vi "Rename Typedefs.vi"(8 "error in (no error)":errorcluster, 11 "ProjectItem in":refnum<class "ProjectItem.lvclass">) -> (0 "error out":errorcluster, 3 "ProjectItem out":refnum<class "ProjectItem.lvclass">)   [LabVIEW 2019, in "ProjectItem.lvclass"]
uses:
  ProjectItem.lvclass
  ProjectItem.lvclass/ProjectItem.ctl
panel:
  out "VI Names":string[](array[string])
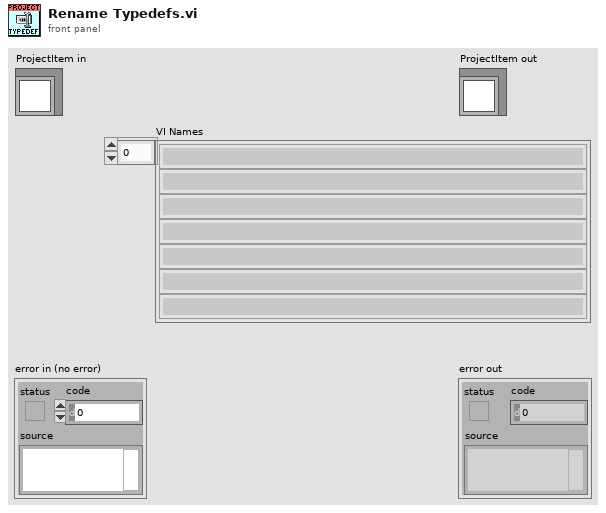
[diagram p1: front panel]
types:
  T1 = cluster{"Class":refnum<vi>, "DynamicVIs":refnum<vi>[], "StaticVIs":refnum<vi>[], "Controls":refnum<vi>[], "Name":string, "Icon":refnum<class "Icon.lvclass">, "Wire Foreground Color":u32}[]
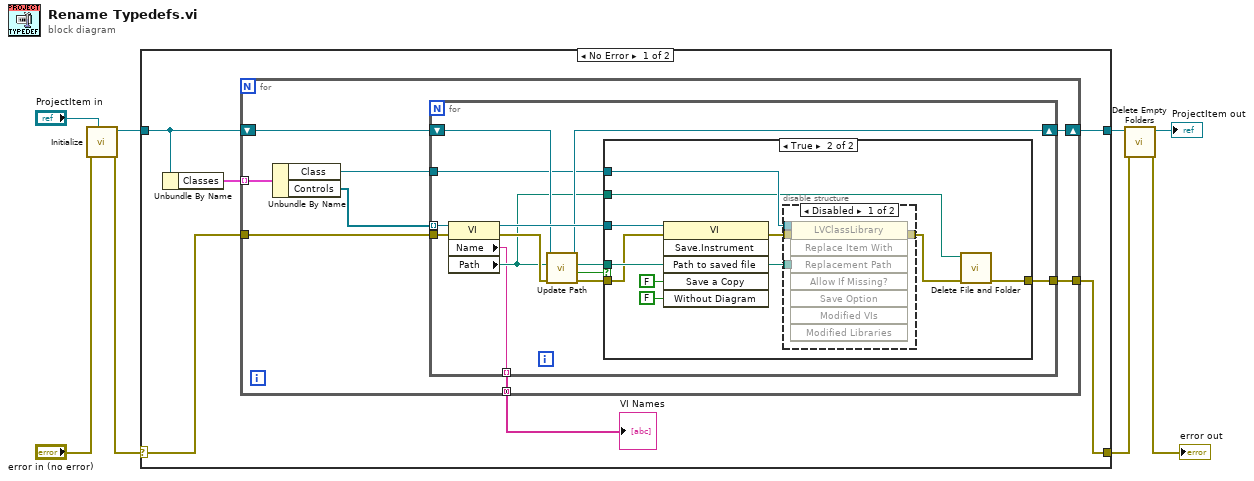
[diagram p0: block diagram]
diagram:
  n1 = call "Initialize.vi"("ProjectItem"="ProjectItem in", "error in (no error)"="error in (no error)") -> ("error out"=w5:errorcluster, "ProjectItem out"=w7:refnum<class "ProjectItem.lvclass">)  [unwired: 8 in]
  n2 = case shown="No Error" w5 {
    selector: w5 -> [w13 w53]
    tunnel: [w10 w53] -> w2
    tunnel: [w14 w52] -> w4
    tunnel: w7 -> [w11 w52]
    frame No Error {
      n3 = Unbundle By Name(w11) -> ("Classes"=w12:T1)
      n4 = for {
        tunnel: w13 -> [w22]
        shift-right: [w21] -> w14
        shift-left: w11 -> [w20]
        tunnel: w12 -> [w19] mode=indexing
        tunnel: [w16] -> w10
        tunnel: [w15] -> w9 mode=concatenating
        n5 = Unbundle By Name(w19) -> ("Class"=w17:refnum<vi>, "Controls"=w18:refnum<vi>[])
        n6 = for {
          tunnel: w22 -> [w32]
          shift-right: [w29] -> w21
          shift-left: w20 -> [w31]
          tunnel: w18 -> [w28] mode=indexing
          tunnel: w17 -> [w27]
          tunnel: [w24] -> w16
          tunnel: [w23] -> w15 mode=indexing
          n7 = property class="VI"(reference=w28, error in=w32) -> (reference out=w35:refnum<vi>, error out=w34:errorcluster, "Name"=w23:string, "Path"=w25:path)
          n8 = call "Update Path.vi"("error in (no error)"=w34, "Path in"=w25, "Rename in"=w31) -> ("error out"=w33:errorcluster, "New Path?"=w26:bool, "Path out"=w30:path, "Rename out"=w29:refnum<class "ProjectItem.lvclass">)  [unwired: 5 in]
          n9 = case shown="True" w26 {
            tunnel: w35 -> [_ w46]
            tunnel: w33 -> [w36 w41]
            tunnel: w30 -> [_ w43]
            tunnel: w27 -> [_ w42]
            tunnel: w25 -> [_ w37]
            tunnel: [w36 w38] -> w24
            frame False {
            }
            frame True {
              n10 = invoke class="VI" method="Save.Instrument"(reference=w46, error in=w41, "Path to saved file"=w43, "Save a Copy"=FALSE, "Without Diagram"=FALSE) -> (error out=w39:errorcluster)  [unwired: 1 in, 5 out]
              n11 = disable-structure shown="Disabled" {
                disable-tunnel: w43 -> [w50 _]
                disable-tunnel: w42 -> [w49 _]
                disable-tunnel: [w48 w51] -> w40
                disable-tunnel: w39 -> [w47 w51]
                frame Disabled {
                  n12 = invoke class="LVClassLibrary" method="Replace Item With"(reference=w49, error in=w47, "Replacement Path"=w50) -> (error out=w48:errorcluster)  [unwired: 5 in, 7 out]
                }
                frame Enabled {
                }
              }
              n13 = call "Delete File and Folder.vi"("error in (no error)"=w40, "Path"=w37) -> ("error out"=w38:errorcluster)  [unwired: 9 in]
            }
          }
        }
      }
      "VI Names" <- w9
    }
    frame Error {
    }
  }
  n14 = call "Delete Empty Folders.vi"("error in (no error)"=w2, "Rename in"=w4) -> ("error out"=→"error out":errorcluster, "Rename out"=→"ProjectItem out":refnum<class "ProjectItem.lvclass">)  [unwired: 8 in]
